vi "DTC.StatusCode.Set.vi"(8 "error in":errorcluster, 11 "Section Ref in":T1 format="%.0x") -> (0 "error out":errorcluster, 3 "Section Ref out":T1 format="%.0x")   [LabVIEW 2019, in "Diagnostics Addon System Explorer.lvlib"]
uses:
  Diagnostics Addon System Explorer.lvlib
  <vilib>/NI VeriStand/Custom Device API/Custom Device Item Ref.ctl
  Types/FG.Action.ctl
  Addon Shared/SubVIs/Constants.vi
  <vilib>/NI/NI VeriStand Advanced SysDef API/SysDef API/SysDef.Property.Set.vi
  <vilib>/NI/NI VeriStand Advanced SysDef API/_SubVIs/SysDef.Property.Set.I32.vi
  <vilib>/NI/NI VeriStand Advanced SysDef API/_SubVIs/SysDef.Property.Set.U32.vi
  <vilib>/NI/NI VeriStand Advanced SysDef API/_SubVIs/SysDef.Property.Set.DBL.Array.vi
  <vilib>/NI/NI VeriStand Advanced SysDef API/_SubVIs/SysDef.Property.Set.String.Array.vi
  <vilib>/NI VeriStand/Custom Device API/NI VeriStand - Get Item Property.vi
  <vilib>/NI VeriStand/Custom Device API/Get Item Property (I32).vi
  <vilib>/NI VeriStand/Custom Device API/Get Item Property (U32).vi
  <vilib>/NI VeriStand/Custom Device API/Get Item Property (Double Array).vi
  <vilib>/NI VeriStand/Custom Device API/Get Item Property (String Array).vi
  <vilib>/NI VeriStand/Custom Device Tools/Custom Device Utility Library/NI VeriStand - Search for All Items by GUID.vi
  <vilib>/NI VeriStand/Custom Device Tools/Custom Device Utility Library/NI VeriStand - Search for Item by Name.vi
  <vilib>/NI VeriStand/Custom Device Tools/Custom Device Utility Library/Custom Device Utility Library.lvlib
  Addon Shared/Diagnostics Addon Shared.lvlib
  <vilib>/NI VeriStand/Custom Device API/Custom Device API.lvlib
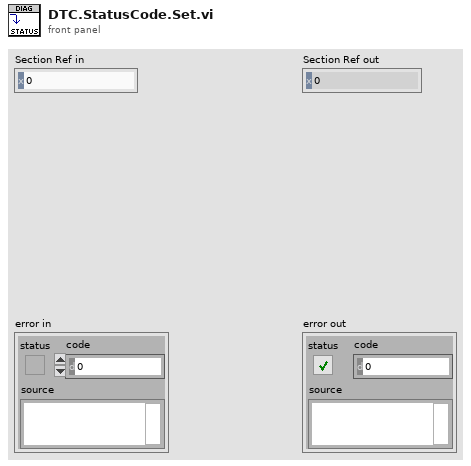
[diagram p1: front panel]
types:
  T1 = typedef "Custom Device API.lvlib/Custom Device Item Ref.ctl" = u64
  T2 = typedef "Diagnostics Addon System Explorer.lvlib/FG.Action.ctl" = enum16{"Get", "Set"}
  T3 = typedef "Diagnostics Addon Shared.lvlib/DTC.Settings.ctl" = cluster{"Descriptor":T4, "Value.Code":dbl[], "Value.String":string[], "Value.J2012String":string[], "Status.Code":dbl[], "Status.String":string[]}
  T4 = typedef "Diagnostics Addon Shared.lvlib/DTC.Descriptor.ctl" = cluster{"DTC Byte Length":i32, "Status Byte Length":i32, "Add Data Byte Length":i32, "Byte Order":enum16{"Motorola", "Intel"}}
  T5 = typedef "Custom Device API.lvlib/Custom Device Item Info.ctl" = cluster{"Name":string, "Is Channel":bool, "GUID":string, "Is Waveform":bool}
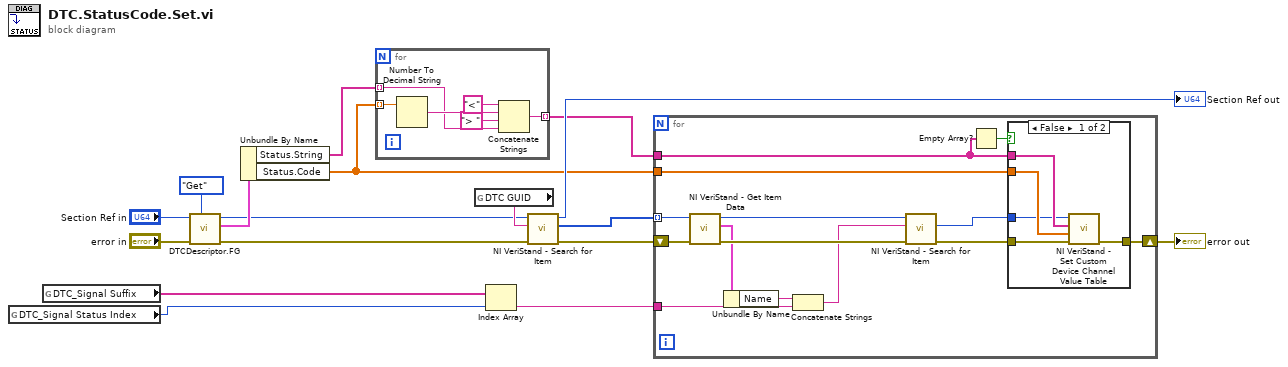
[diagram p0: block diagram]
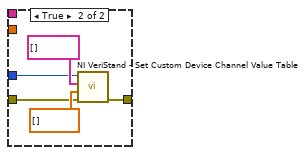
[diagram p2: hidden frame]
diagram:
  n1 = global read "Constants.vi" "DTC_Signal Status Index"() -> (w10:i32)
  n2 = global read "Constants.vi" "DTC_Signal Suffix"() -> (w16:string[])
  n3 = call "DTCDescriptor.FG.vi"("Action"=FG.Action."Get", "error in (no error)"="error in", "Device Item Ref in"="Section Ref in") -> ("error out"=w6:errorcluster, "DTC descriptor"=w8:T3, "Device Item Ref out"=w4:T1)  [unwired: 6 in]
  n4 = Unbundle By Name(w8) -> ("Status.String"=w2:string[], "Status.Code"=w3:dbl[])
  n5 = for {
    tunnel: w2 -> [w19] mode=indexing
    tunnel: w3 -> [w20] mode=indexing
    tunnel: [w18] -> w1 mode=indexing
    n6 = Number To Decimal String(number=w20) -> (decimal integer string=w21:string)  [unwired: 1 in]
    n7 = Concatenate Strings("<" ("string"), w21, "> " ("string"), w19) -> (w18:string)
  }
  n8 = global read "Constants.vi" "DTC GUID"() -> (w17:string)
  n9 = Index Array(array=w16, index=w10) -> (element=w13:string)
  n10 = call-poly <vilib>:"NI VeriStand - Search for Item.vi"("error in"=w6, "Item GUID"=w17, "Section Ref in"=w4) -> ("error out"=w15:errorcluster, "Item Refs"=w14:T1[], "Section Ref out"=→"Section Ref out":T1)  [unwired: 5 in, 1 out]
  n11 = for {
    shift-right: [w34] -> w12
    shift-left: w15 -> [w29]
    tunnel: w14 -> [w31] mode=indexing
    tunnel: w13 -> [w25]
    tunnel: w1 -> [w33]
    tunnel: w3 -> [w32]
    n12 = call <vilib>:"NI VeriStand - Get Item Data.vi"("error in (no error)"=w29, "Item Ref in"=w31) -> ("error out"=w28:errorcluster, "Item Info"=w27:T5, "Item Ref out"=w30:T1)  [unwired: 6 in, 1 out]
    n13 = Unbundle By Name(w27) -> ("Name"=w26:string)
    n14 = Concatenate Strings(w26, w25) -> (w24:string)
    n15 = call-poly <vilib>:"NI VeriStand - Search for Item.vi"("error in"=w28, "Item Name"=w24, "Section Ref in"=w30) -> ("error out"=w35:errorcluster, "Item Ref"=w36:T1)  [unwired: 5 in, 2 out]
    n16 = Empty Array?(array=w33) -> (empty?=w37:bool)
    n17 = case shown="False" w37 {
      tunnel: w33 -> [w42 _]
      tunnel: w32 -> [w41 _]
      tunnel: [w40 w47] -> w34
      tunnel: w36 -> [w38 w44]
      tunnel: w35 -> [w39 w43]
      frame False {
        n18 = call <vilib>:"NI VeriStand - Set Custom Device Channel Value Table.vi"("error in (no error)"=w39, "Values"=w41, "Names"=w42, "Channel Ref in"=w38) -> ("error out"=w40:errorcluster)  [unwired: 6 in, 1 out]
      }
      frame True {
        n19 = call <vilib>:"NI VeriStand - Set Custom Device Channel Value Table.vi"("error in (no error)"=w43, "Values"=dbl[] [], "Names"=string[] [], "Channel Ref in"=w44) -> ("error out"=w47:errorcluster)  [unwired: 6 in, 1 out]
      }
    }
  }
  "error out" <- w12
